vi "VC_UItem.vi"(8 "error in (no error)":errorcluster, 10 "UI Item label":string, 11 "UI_Actor in":refnum<class "UI_Actor.lvclass">) -> (0 "error out":errorcluster, 3 "UI_Actor out":refnum<class "UI_Actor.lvclass">)   [LabVIEW 2020, in "UI_Actor.lvlib" / "UI_Actor.lvclass"]
doc: "Ce VI sert à mutualiser le catch des value changes de l'UI dans l'acteur. Pour cela:\n- placer son send dans la UE loop, dans les cas qui interressent (mutulaliser BG avec un reg event sur la liste des sources), et cabler le label.\n- overrider le VI pour gérer la réaction. Utiliser ici le polymorph UI Access pour un max d'efficacité."
uses:
  UI_Actor.lvclass
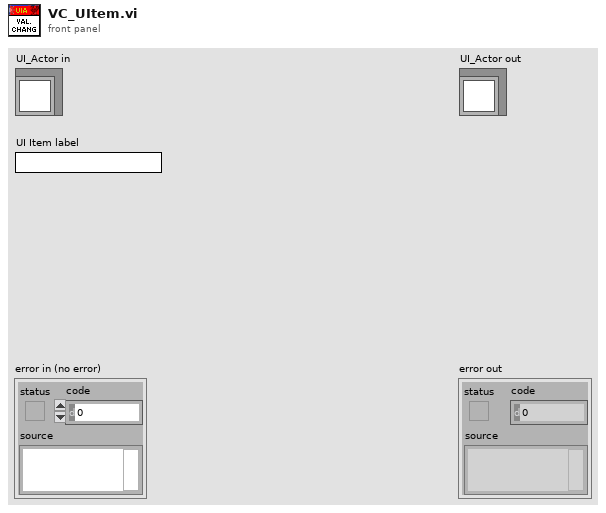
[diagram p1: front panel]
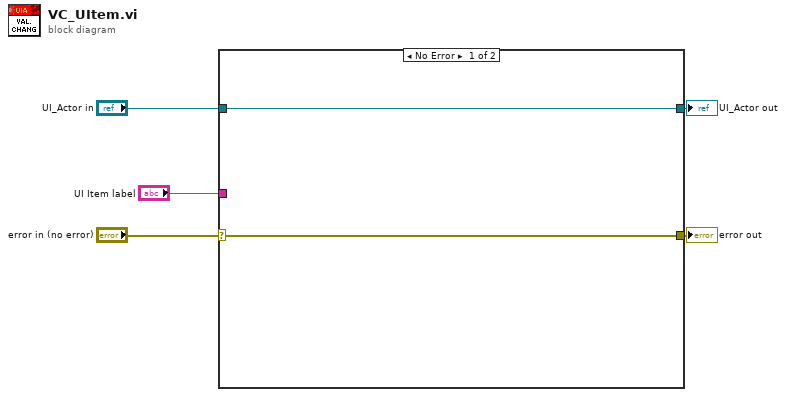
[diagram p0: block diagram]
diagram:
  n1 = case shown="No Error" "error in (no error)" {
    selector: "error in (no error)" -> [w6 w9]
    tunnel: [w6 w9] -> w4
    tunnel: [w7 w8] -> w2
    tunnel: "UI_Actor in" -> [w7 w8]
    tunnel: "UI Item label" -> [_ _]
    frame No Error {
    }
    frame Error {
    }
  }
  "error out" <- w4
  "UI_Actor out" <- w2
